vi "VINode_Create.vi"(0 "reference in":refnum<class "VINode.lvclass">, 5 "error in (no error)":errorcluster) -> (14 "reference out":refnum<class "VINode.lvclass">, 19 "error out":errorcluster)   [LabVIEW 2016, in "VINode.lvclass"]
doc: "Creates and initializes a new ClassNode object.\n\nThis object should be destroyed using a ClassNode destructor VI or a virtual base class destructor VI.\n\n[GOOP 2.1]"
uses:
  <resource>/Framework/Providers/Open_GDS/UML/VINode_class/VINode.lvclass
  C:/Program Files (x86)/National Instruments/LabVIEW 2016/resource/Framework/Providers/Open_GDS/UML/RectangularNode_class/RectangularNode.lvclass
  <resource>/Framework/Providers/Open_GDS/UML/MultiLineString_class/SizeType.ctl
  <resource>/Framework/Providers/Open_GDS/UML/General/Rectangle/Rectangle Rectangle2D.ctl
  <resource>/Framework/Providers/Open_GDS/UML/MultiLineString_class/JustificationType.ctl
  <resource>/Framework/Providers/Open_GDS/UML/RectangularNode_class/RectangularNode.lvclass
  <resource>/Framework/Providers/Open_GDS/UML/MultiLineString_class/MultiLineString.lvclass
panel:
  # "The input reference should only\nbe wired when this method is called\nby a sub class constructor."
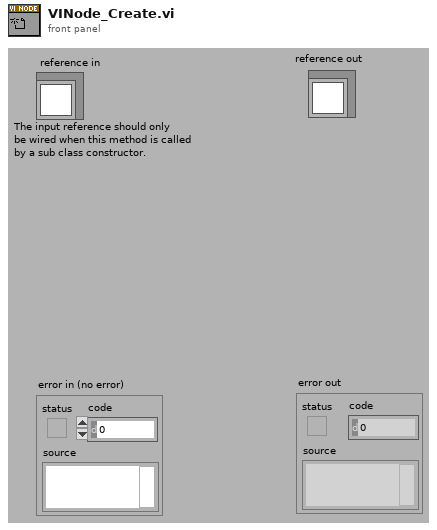
[diagram p1: front panel]
types:
  T1 = typedef "MultiLineString.lvclass/JustificationType.ctl" = enum16{"LEFT", "CENTER", "RIGHT"}
  T2 = typedef "Rectangle Rectangle2D.ctl" = cluster{"x":dbl, "y":dbl, "width":dbl, "height":dbl}
  T3 = typedef "MultiLineString.lvclass/SizeType.ctl" = enum16{"LARGE", "NORMAL", "SMALL"}
  T4 = typedef "VINode.lvclass/ObjectAttributes.ctl" = cluster{"midHeight":dbl, "botHeight":dbl, "Name":refnum<class "MultiLineString.lvclass">, "DEFAULT_COMPARTMENT_HEIGHT":i32, "DEFAULT_WIDTH":i32, "DEFAULT_HEIGHT":i32, "VIPath":path, "Description":refnum<class "MultiLineString.lvclass">, "ShowDescription":bool}
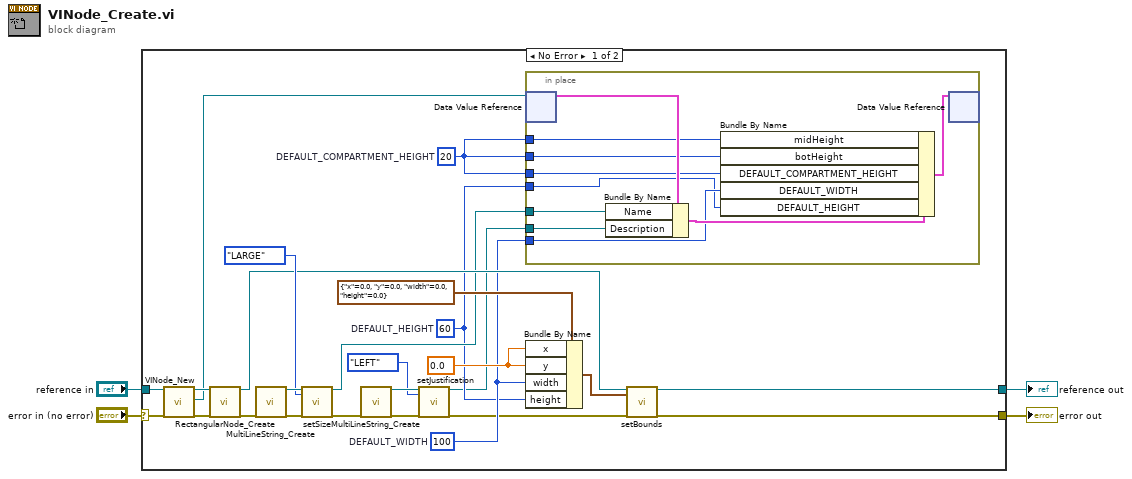
[diagram p0: block diagram]
diagram:
  n1 = case shown="No Error" "error in (no error)" {
    selector: "error in (no error)" -> [w29 w41]
    tunnel: [w12 w40] -> w4
    tunnel: [w11 w41] -> w3
    tunnel: "reference in" -> [w28 w40]
    frame No Error {
      w18 = 0.0 ("x")
      w14 = 60  # DEFAULT_HEIGHT
      w15 = 100  # DEFAULT_WIDTH
      w16 = 20  # DEFAULT_COMPARTMENT_HEIGHT
      n2 = call <resource>:"VINode_New.vi"("reference in"=w28, "error in (no error)"=w29) -> ("reference out"=w26:refnum<class "VINode.lvclass">, "DVRRefOut"=w13:refnum<data-value>, "error out"=w27:errorcluster)  [unwired: 2 in, 13 out]
      n3 = call <resource>:"RectangularNode_Create.vi"("reference"=w26, "error in (no error)"=w27) -> ("reference out"=w21:refnum<class "VINode.lvclass">, "error out"=w25:errorcluster)  [unwired: 1 in, 15 out]
      n4 = call <resource>:"MultiLineString_Create.vi"("error in (no error)"=w25) -> ("reference out"=w24:refnum<class "MultiLineString.lvclass">, "error out"=w23:errorcluster)  [unwired: 2 in, 15 out]
      n5 = call <resource>:"setSize.vi"("reference"=w24, "size"=SizeType."LARGE", "error in (no error)"=w23) -> ("reference out"=w17:refnum<class "MultiLineString.lvclass">, "error out"=w7:errorcluster)  [unwired: 15 out]
      n6 = call <resource>:"MultiLineString_Create.vi"("error in (no error)"=w7) -> ("reference out"=w10:refnum<class "MultiLineString.lvclass">, "error out"=w9:errorcluster)  [unwired: 2 in, 15 out]
      n7 = call <resource>:"setJustification.vi"("reference"=w10, "justification"=JustificationType."LEFT", "error in (no error)"=w9) -> ("reference out"=w5:refnum<class "MultiLineString.lvclass">, "error out"=w6:errorcluster)  [unwired: 15 out]
      n8 = in-place {
        in-place-border: w17 -> [w38]
        in-place-border: w16 -> [w36]
        in-place-border: w16 -> [w35]
        in-place-border: w16 -> [w34]
        in-place-border: w15 -> [w33]
        in-place-border: w14 -> [w32]
        in-place-border: w5 -> [w30]
        n9 = in-place-dvr #1(w13) -> (w39:T4)  [unwired: 1 out]
        n10 = Bundle By Name(cluster=w39, "Name"=w38, "Description"=w30) -> (w37:T4)
        n11 = Bundle By Name(cluster=w37, "midHeight"=w36, "botHeight"=w35, "DEFAULT_COMPARTMENT_HEIGHT"=w34, "DEFAULT_WIDTH"=w33, "DEFAULT_HEIGHT"=w32) -> (w31:T4)
        n12 = in-place-dvr #1(w31) -> ()  [unwired: 2 out]
      }
      n13 = Bundle By Name(cluster=T2 {"x"=0.0, "y"=0.0, "width"=0.0, "height"=0.0} ("bounds"), "x"=w18, "y"=w18, "width"=w15, "height"=w14) -> (w20:T2)
      n14 = call-dynamic "setBounds.vi"("reference"=w21, "bounds"=w20, "error in (no error)"=w6) -> ("reference out"=w12:refnum<class "VINode.lvclass">, "error out"=w11:errorcluster)  [unwired: 15 in]
    }
    frame Error {
    }
  }
  "error out" <- w3
  "reference out" <- w4
